vi "report page.vi"() -> (2 "This VI":refnum<vi>)   [LabVIEW 2019]
uses:
  <vilib>/addons/database/NI_Database_API.lvlib
  <vilib>/addons/database/_DB Variant To Data/Database Variant To Data.xnode
  <vilib>/addons/database/Connection.llb/DB Tools Open Connec (String).vi
  <vilib>/Utility/NIReport.llb/NI_report.lvclass
  <vilib>/Utility/NIReport.llb/Append Text Table to Report (wrap).vi
  <vilib>/Utility/miscctls.llb/LVRowAndColumnTypeDef.ctl
panel:
  out "show img error":errorcluster
  in  "show":bool
  out "Selection Start":T1
  in  "stop":bool
  out "Cancel Button 2":bool
  out "Column Header Strings[]":string[](array[string])=["pallet_num", "date_time", "Grate Bar Defect", "Curvature", "SWL_sen", "SWR_sen", "SWL_cam", "SWR_cam", "def_Type", "grtbr_situation"]
  out "error out":errorcluster
  in  "curv-sit":u16(ring) items=["normal", "critical"]
  in  "curv-sit":bool
  in  "SWR-cam":u16(ring) items=["yes", "no"]
  in  "SWR-cam":bool
  in  "SWL-cam":u16(ring) items=["yes", "no"]
  in  "SWL-cam":bool
  in  "SWR-sen":u16(ring) items=["yes", "no"]
  in  "SWR_sen":bool
  in  "SWL-sen":u16(ring) items=["yes", "no"]
  in  "SWL-sen":bool
  out "Report":string
  in  "Cancel Button":bool
  out "Time":string="2019/01/29   15:25:26"
  in  "Pallet Sit":u16(ring) items=["normal", "warning", "critical"]
  in  "Defect":u16(ring) items=["Type 1", "Type 2", "Type 3"]
  in  "Pallet Num":u16=1 min=1 max=260 step=1
  in  "Time Select":u16(ring) items=["Selected Period", "Last Day", "Last Week", "Last Month"]
  in  "From":timestamp=timestamp(3613783866.3658285 s since 1904-01-01) format="%<%X\n%d/%m/%Y>T"
  in  "Until":timestamp=timestamp(3613750200 s since 1904-01-01) format="%<%X\n%d/%m/%Y>T"
  in  "Pallet_Situation":bool
  in  "Defect Type":bool
  in  "Pallet Number 2":bool
  in  "Time 2":bool
  in  "Save Button":bool
  in  "Query":bool caption="Reset Signal"
  in  "error in":errorcluster
  out "error out 2":errorcluster
  out "Table":string[][](table)
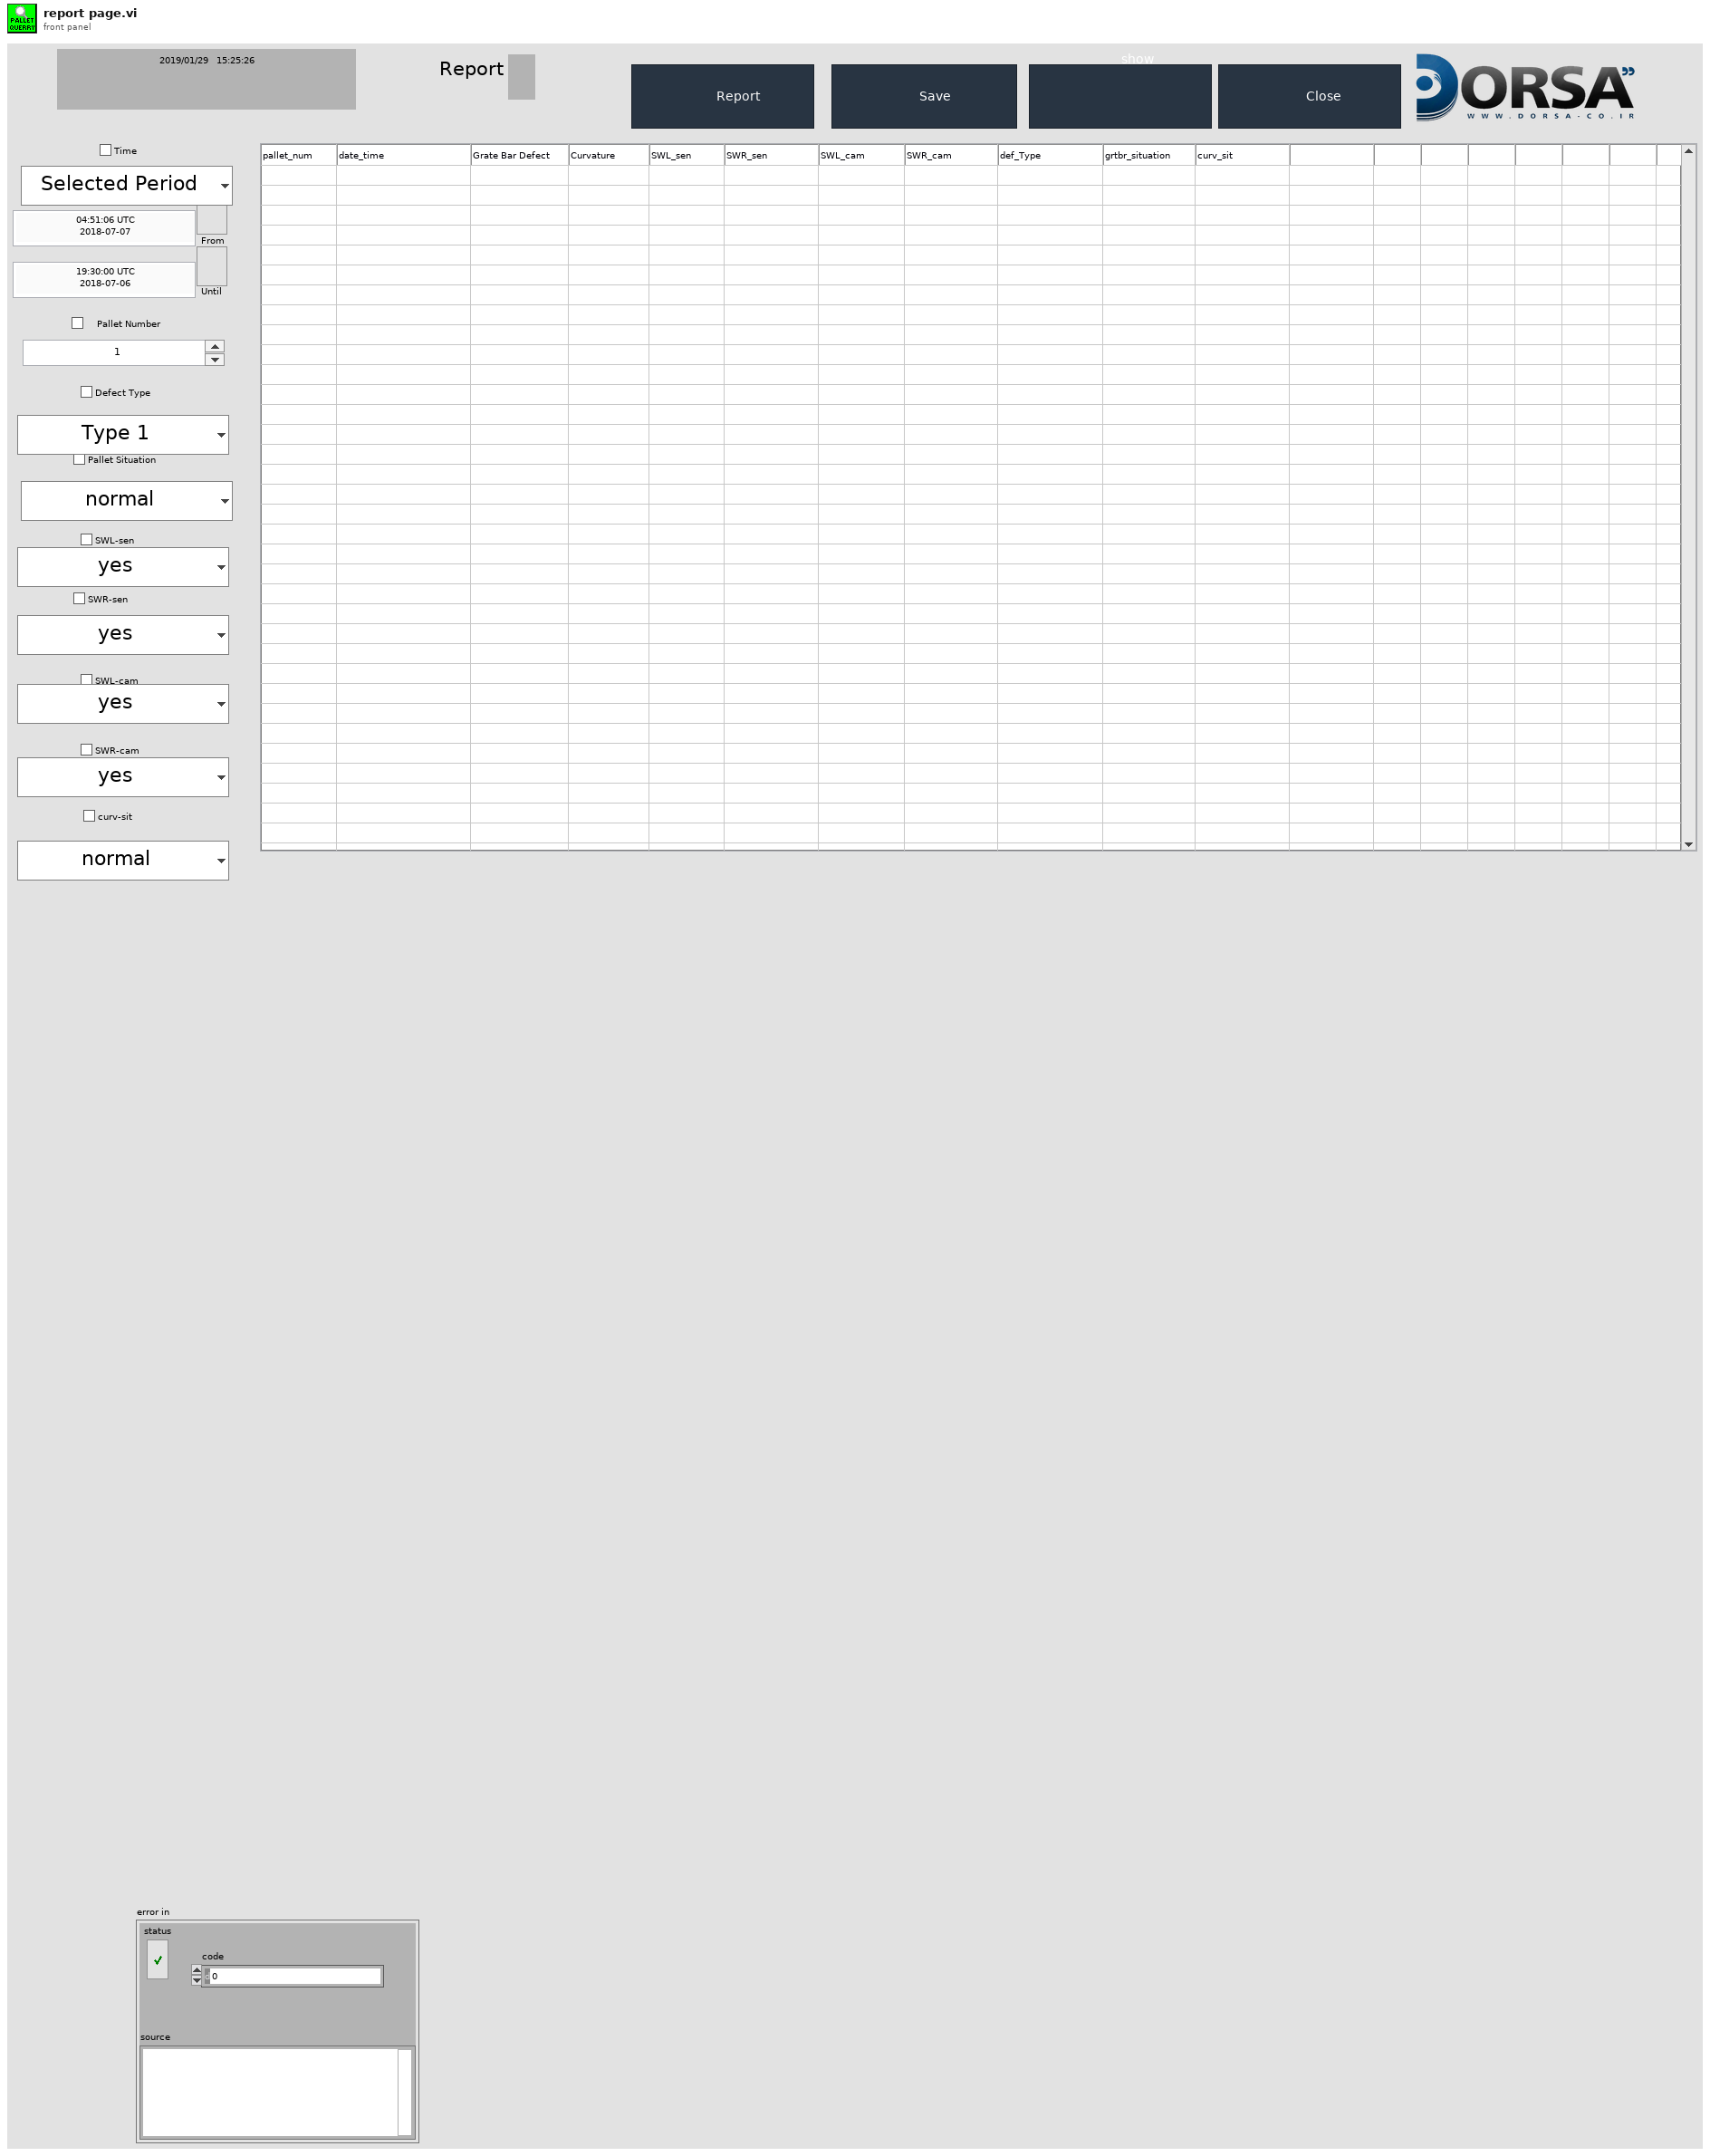
[diagram p1: front panel]
types:
  T1 = typedef "LVRowAndColumnTypeDef.ctl" = cluster{"Row":i32, "Column":i32}
  T2 = typedef "Image Type" = u32
  T3 = enum16{"Standard Report", "HTML", "Word", "Excel"}
  T4 = typedef "NI_Database_API.lvlib/Conn ObjectReference.ctl" = refnum<k1>
  T5 = typedef "IMAQ Image.ctl" = refnum<image>
  T6 = enum32{"Invalid", "Standard", "Closed", "Hidden", "Minimized", "Maximized"}
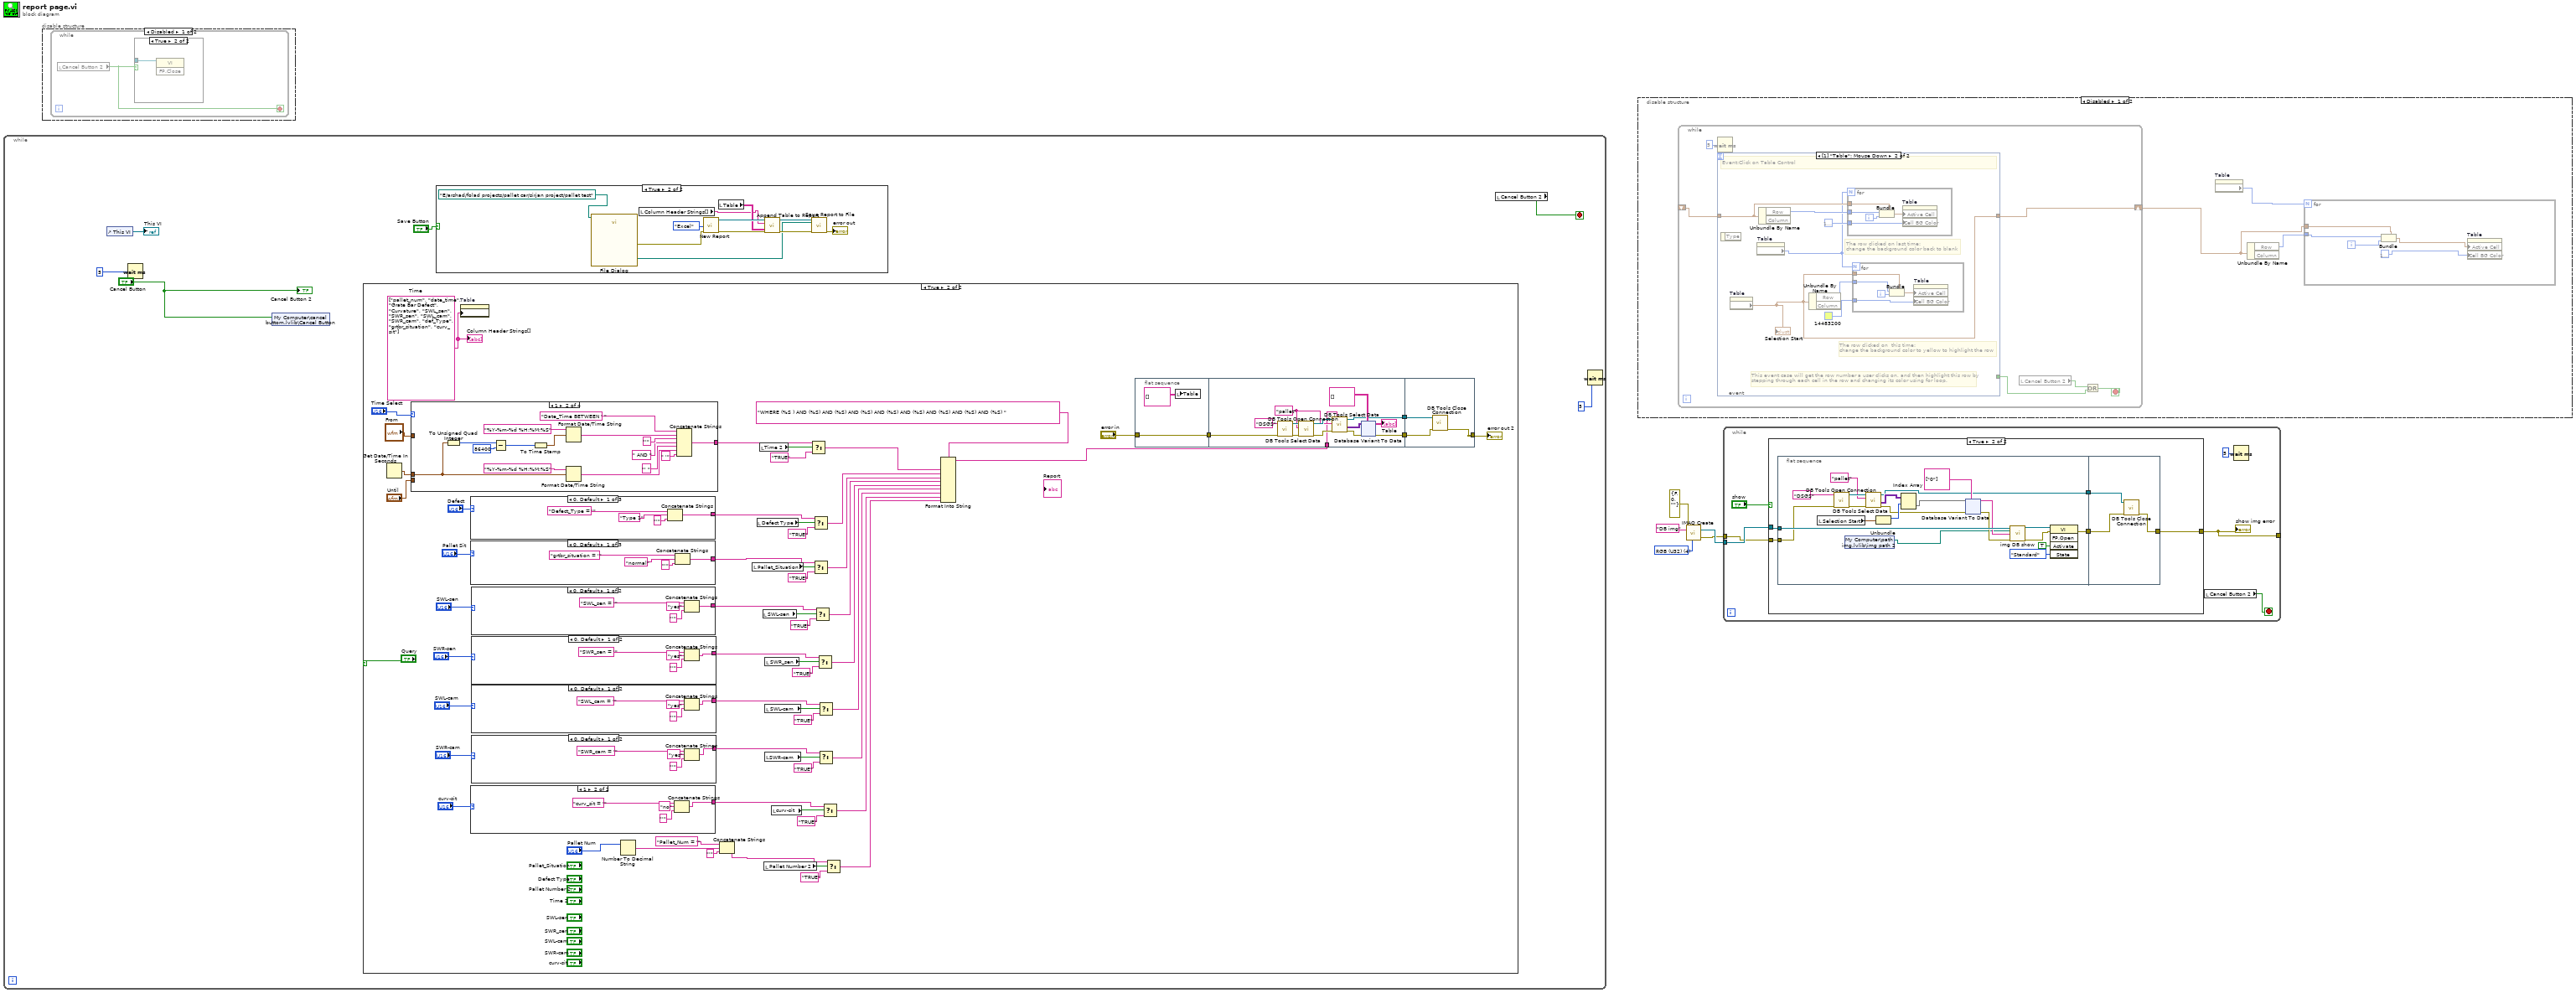
[diagram p0: block diagram]
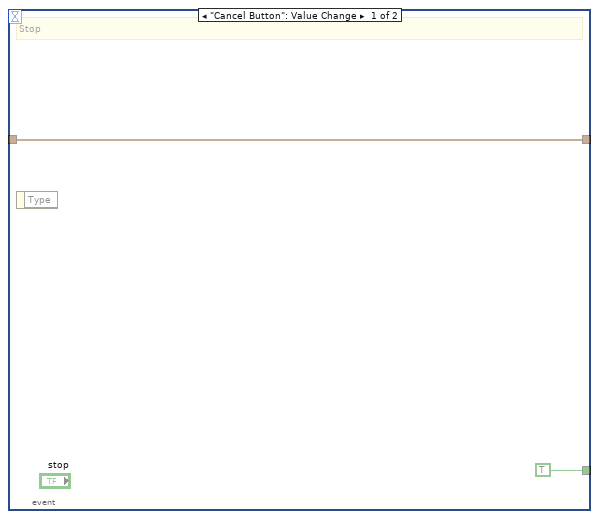
[diagram p2: hidden frame]
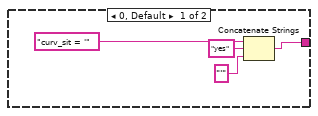
[diagram p8: hidden frame]
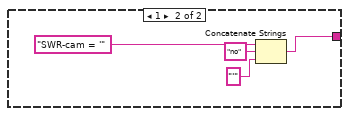
[diagram p9: hidden frame]
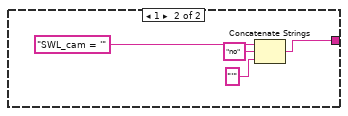
[diagram p10: hidden frame]
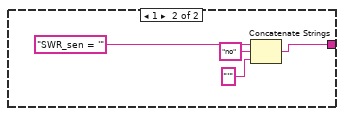
[diagram p11: hidden frame]
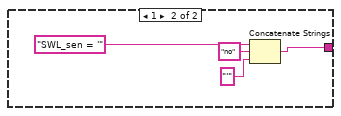
[diagram p12: hidden frame]
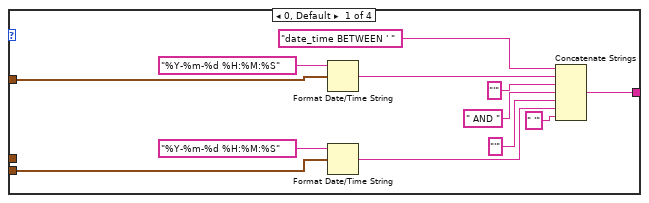
[diagram p13: hidden frame]
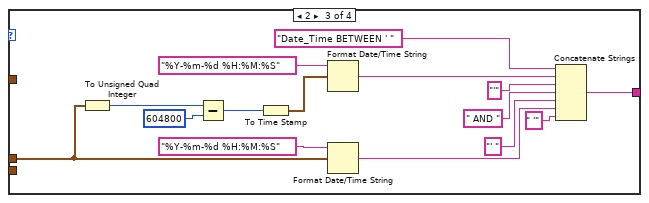
[diagram p14: hidden frame]
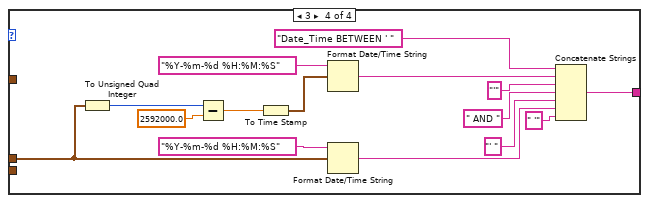
[diagram p15: hidden frame]
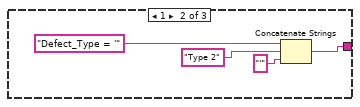
[diagram p16: hidden frame]
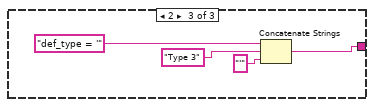
[diagram p17: hidden frame]
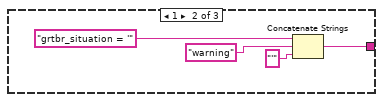
[diagram p18: hidden frame]
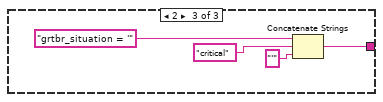
[diagram p19: hidden frame]
diagram:
  w1 = T2 4 items=["Grayscale (U8)", "Grayscale (I16)", "Grayscale (SGL)", "Complex (CSG)", "RGB (U32)", "HSL (U32)", "RGB (U64)", "Grayscale (U16)"] ("Image Type")
  n1 = while {
    stop <- w11 stop-if-true
    n2 = control-ref of="This VI"() -> (→"This VI":refnum<vi>)
    n3 = Wait (ms)(milliseconds to wait=u32 5) -> ()  [unwired: 1 out]
    n4 = shared-variable "My Computer\\cancel buttom.lvlib\\Cancel Button"("Cancel Button") -> ()  [unwired: 1 in, 1 out]
    n5 = case shown="True" "Query" {
      frame False {
      }
      frame True {
        w26 = string[] ["pallet_num", "date_time", "Grate Bar Defect", "Curvature", "SWL_sen", "SWR_sen", "SWL_cam", "SWR_cam", "def_Type", "grtbr_situation", "curv_sit"] ("Column Header Strings[]")
        n6 = Get Date/Time In Seconds() -> (seconds since 1Jan1904=w73:timestamp)
        n7 = case shown="1" "Time Select" {
          tunnel: "From" -> [w193 _ _ _]
          tunnel: "Until" -> [w191 _ _ _]
          tunnel: [w186 w200 w213 w228] -> w74
          tunnel: w73 -> [_ w198 w215 w230]
          frame 0, Default {
            n8 = Format Date/Time String(time format string (%c)="%Y-%m-%d %H:%M:%S", seconds (now)=w193) -> (date/time string=w192:string)  [unwired: 1 in]
            n9 = Format Date/Time String(time format string (%c)="%Y-%m-%d %H:%M:%S", seconds (now)=w191) -> (date/time string=w188:string)  [unwired: 1 in]
            n10 = Concatenate Strings("date_time BETWEEN ' " ("condition"), w192, "'" ("condition"), " AND " ("time format string (%c)"), "'" ("string"), w188, " '" ("string")) -> (w186:string)
          }
          frame 1 {
            n11 = To Unsigned Quad Integer(1:w198) -> (0:w210:u64)
            n12 = Subtract(x=w210, y=u64 86400) -> (x-y=w212:u64)
            n13 = To Time Stamp(1:w212) -> (0:w199:timestamp)
            n14 = Format Date/Time String(time format string (%c)="%Y-%m-%d %H:%M:%S", seconds (now)=w199) -> (date/time string=w205:string)  [unwired: 1 in]
            n15 = Format Date/Time String(time format string (%c)="%Y-%m-%d %H:%M:%S", seconds (now)=w198) -> (date/time string=w202:string)  [unwired: 1 in]
            n16 = Concatenate Strings("Date_Time BETWEEN ' " ("condition"), w205, "'" ("condition"), " AND " ("time format string (%c)"), "' " ("string"), w202, " '" ("string")) -> (w200:string)
          }
          frame 2 {
            n17 = To Unsigned Quad Integer(1:w215) -> (0:w218:u64)
            n18 = Subtract(x=w218, y=u64 604800) -> (x-y=w216:u64)
            n19 = To Time Stamp(1:w216) -> (0:w214:timestamp)
            n20 = Format Date/Time String(time format string (%c)="%Y-%m-%d %H:%M:%S", seconds (now)=w214) -> (date/time string=w223:string)  [unwired: 1 in]
            n21 = Format Date/Time String(time format string (%c)="%Y-%m-%d %H:%M:%S", seconds (now)=w215) -> (date/time string=w220:string)  [unwired: 1 in]
            n22 = Concatenate Strings("Date_Time BETWEEN ' " ("condition"), w223, "'" ("condition"), " AND " ("time format string (%c)"), "' " ("string"), w220, " '" ("string")) -> (w213:string)
          }
          frame 3 {
            n23 = To Unsigned Quad Integer(1:w230) -> (0:w232:u64)
            n24 = Subtract(x=w232, y=2592000.0) -> (x-y=w233:dbl)
            n25 = To Time Stamp(1:w233) -> (0:w229:timestamp)
            n26 = Format Date/Time String(time format string (%c)="%Y-%m-%d %H:%M:%S", seconds (now)=w229) -> (date/time string=w238:string)  [unwired: 1 in]
            n27 = Format Date/Time String(time format string (%c)="%Y-%m-%d %H:%M:%S", seconds (now)=w230) -> (date/time string=w241:string)  [unwired: 1 in]
            n28 = Concatenate Strings("Date_Time BETWEEN ' " ("condition"), w238, "'" ("condition"), " AND " ("time format string (%c)"), "' " ("string"), w241, " '" ("string")) -> (w228:string)
          }
        }
        n29 = property on="Table" class="Tbl (strict)"("Column Headers[]"=w26) -> ()  [unwired: 2 in, 2 out]
        n30 = case shown="0, Default" "Defect" {
          tunnel: [w243 w247 w251] -> w76
          frame 0, Default {
            n31 = Concatenate Strings("Defect_Type = '" ("string"), "Type 1" ("string"), "'" ("string")) -> (w243:string)
          }
          frame 1 {
            n32 = Concatenate Strings("Defect_Type = '" ("string"), "Type 2" ("string"), "'" ("string")) -> (w247:string)
          }
          frame 2 {
            n33 = Concatenate Strings("def_type = '" ("string"), "Type 3" ("string"), "'" ("string")) -> (w251:string)
          }
        }
        n34 = case shown="0, Default" "Pallet Sit" {
          tunnel: [w255 w259 w263] -> w77
          frame 0, Default {
            n35 = Concatenate Strings("grtbr_situation = '" ("string"), "normal" ("string"), "'" ("string")) -> (w255:string)
          }
          frame 1 {
            n36 = Concatenate Strings("grtbr_situation = '" ("string"), "warning" ("string"), "'" ("string")) -> (w259:string)
          }
          frame 2 {
            n37 = Concatenate Strings("grtbr_situation = '" ("string"), "critical" ("string"), "'" ("string")) -> (w263:string)
          }
        }
        n38 = case shown="1" "curv-sit" {
          tunnel: [w146 w150] -> w55
          frame 0, Default {
            n39 = Concatenate Strings("curv_sit = '" ("string"), "yes" ("string"), "'" ("string")) -> (w146:string)
          }
          frame 1 {
            n40 = Concatenate Strings("curv_sit = '" ("string"), "no" ("string"), "'" ("string")) -> (w150:string)
          }
        }
        n41 = case shown="0, Default" "SWL-sen" {
          tunnel: [w178 w182] -> w59
          frame 0, Default {
            n42 = Concatenate Strings("SWL_sen = '" ("string"), "yes" ("string"), "'" ("string")) -> (w178:string)
          }
          frame 1 {
            n43 = Concatenate Strings("SWL_sen = '" ("string"), "no" ("string"), "'" ("string")) -> (w182:string)
          }
        }
        n44 = case shown="0, Default" "SWR-sen" {
          tunnel: [w170 w174] -> w58
          frame 0, Default {
            n45 = Concatenate Strings("SWR_sen = '" ("string"), "yes" ("string"), "'" ("string")) -> (w170:string)
          }
          frame 1 {
            n46 = Concatenate Strings("SWR_sen = '" ("string"), "no" ("string"), "'" ("string")) -> (w174:string)
          }
        }
        n47 = case shown="0, Default" "SWL-cam" {
          tunnel: [w162 w166] -> w57
          frame 0, Default {
            n48 = Concatenate Strings("SWL_cam = '" ("string"), "yes" ("string"), "'" ("string")) -> (w162:string)
          }
          frame 1 {
            n49 = Concatenate Strings("SWL_cam = '" ("string"), "no" ("string"), "'" ("string")) -> (w166:string)
          }
        }
        n50 = case shown="0, Default" "SWR-cam" {
          tunnel: [w154 w158] -> w56
          frame 0, Default {
            n51 = Concatenate Strings("SWR_cam = '" ("string"), "yes" ("string"), "'" ("string")) -> (w154:string)
          }
          frame 1 {
            n52 = Concatenate Strings("SWR-cam = '" ("string"), "no" ("string"), "'" ("string")) -> (w158:string)
          }
        }
        n53 = Number To Decimal String(number="Pallet Num") -> (decimal integer string=w81:string)  [unwired: 1 in]
        n54 = Concatenate Strings("Pallet_Num = '" ("string"), w81, "'" ("string")) -> (w75:string)
        n55 = local read "Pallet_Situation"() -> (w50:bool)
        n56 = local read "Defect Type"() -> (w51:bool)
        n57 = local read "Time 2"() -> (w54:bool)
        n58 = local read "SWL-sen"() -> (w47:bool)
        n59 = local read "Pallet Number 2"() -> (w38:bool)
        n60 = local read "SWR-cam"() -> (w42:bool)
        n61 = local read "SWR_sen"() -> (w46:bool)
        n62 = local read "SWL-cam"() -> (w43:bool)
        n63 = local read "curv-sit"() -> (w39:bool)
        n64 = Select(t=w74, s=w54, f="TRUE") -> (s? t:f=w36:string)
        n65 = Select(t=w76, s=w51, f="TRUE") -> (s? t:f=w35:string)
        n66 = Select(t=w77, s=w50, f="TRUE") -> (s? t:f=w34:string)
        n67 = Select(t=w59, s=w47, f="TRUE") -> (s? t:f=w33:string)
        n68 = Select(t=w58, s=w46, f="TRUE") -> (s? t:f=w32:string)
        n69 = Select(t=w57, s=w43, f="TRUE") -> (s? t:f=w31:string)
        n70 = Select(t=w56, s=w42, f="TRUE") -> (s? t:f=w30:string)
        n71 = Select(t=w55, s=w39, f="TRUE") -> (s? t:f=w29:string)
        n72 = Select(t=w75, s=w38, f="TRUE") -> (s? t:f=w28:string)
        n73 = Format Into String(format string="WHERE (%S ) AND (%S) AND (%S) AND (%S) AND (%S) AND (%S) AND (%S) AND (%S) AND (%S) ", w36, w35, w34, w33, w32, w31, w30, w29, w28) -> (resulting string=w78:string)  [unwired: 2 in, 1 out]
        n74 = flat-sequence {
          tunnel: [w83] -> w82
          tunnel: "error in" -> [w83]
          tunnel: w82 -> [w96]
          tunnel: w78 -> [w85]
          tunnel: [w91] -> w25
          tunnel: [w86] -> w24
          tunnel: [w143] -> w71
          tunnel: w25 -> [w144]
          tunnel: w24 -> [w145]
          frame #0 {
            n75 = local write "Table"(string[][] []) -> ()
          }
          frame #1 {
            w88 = "pallet" ("table name")
            n76 = call-poly <vilib>:"DB Tools Open Connection.vi"("error in (no error)"=w96, "connection information"="DSGS" ("Database")) -> ("error out"=w95:errorcluster, "connection reference"=w94:T4)  [unwired: 6 in]
            n77 = call <vilib>:"DB Tools Select Data.vi"("error in (no error)"=w95, "table"=w88, "connection reference"=w94) -> ("error out"=w93:errorcluster, "connection reference out"=w92:T4)  [unwired: 3 in, 1 out]
            n78 = call <vilib>:"DB Tools Select Data.vi"("condition"=w85, "error in (no error)"=w93, "table"=w88, "connection reference"=w92) -> ("error out"=w98:errorcluster, "data"=w97:variant[][], "connection reference out"=w86:T4)  [unwired: 2 in]
            n79 = xnode "Database Variant To Data"("database variant"=w97, "error in (no error)"=w98, "type"=string[][] []) -> ("data"=→"Table":string[][], "error out"=w91:errorcluster)
          }
          frame #2 {
            n80 = call <vilib>:"DB Tools Close Connection.vi"("error in (no error)"=w144, "connection reference"=w145) -> ("error out"=w143:errorcluster)  [unwired: 5 in]
          }
        }
        "error out 2" <- w71
        "Column Header Strings[]" <- w26
      }
    }
    n81 = case shown="True" "Save Button" {
      frame False {
      }
      frame True {
        n82 = call "File Dialog"("start path"=path "E:/arshad/folad projects/pallet car/sirjan project/pallet test" ("report file path")) -> ("selected path"=w14:path, "error out"=w13:errorcluster)  [unwired: 11 in, 2 out]
        n83 = local read "Column Header Strings[]"() -> (w16:string[])
        n84 = call <vilib>:"New Report.vi"("report type"=T3."Excel", "error in (no error)"=w13) -> ("report out"=w22:refnum<class "NI_report.lvclass">, "error out"=w21:errorcluster)  [unwired: 12 in]
        n85 = local read "Table"() -> (w20:string[][])
        n86 = call-poly <vilib>:"Append Table to Report.vi"("report in"=w22, "column headers"=w16, "text data"=w20, "error in (no error)"=w21) -> ("report out"=w19:refnum<class "NI_report.lvclass">, "error out"=w18:errorcluster)  [unwired: 8 in, 2 out]
        n87 = call-dynamic "Save Report to File.vi"("report in"=w19, "report file path"=w14, "error in (no error)"=w18) -> ("error out"=→"error out":errorcluster)  [unwired: 11 in, 1 out]
      }
    }
    n88 = local read "Cancel Button 2"() -> (w11:bool)
    n89 = Wait (ms)(milliseconds to wait=u32 5) -> ()  [unwired: 1 out]
    "Cancel Button 2" <- "Cancel Button"
  }
  n90 = disable-structure shown="Disabled" {
    frame Disabled {
      n91 = while {
        stop <- w268 stop-if-true
        n92 = local read "Cancel Button 2"() -> (w268:bool)
        n93 = case shown="True" w268 {
          tunnel: [_ w269] -> w267
          frame False {
          }
          frame True {
            n94 = invoke class="VI" method="FP.Close"(reference=w269) -> ()  [unwired: 2 in, 3 out]
          }
        }
      }
    }
    frame Enabled {
    }
  }
  n95 = disable-structure shown="Disabled" {
    frame Disabled {
      n96 = while {
        shift-right: [w281] -> w270
        shift-left: _ -> [w282]
        stop <- w278 stop-if-true
        n97 = event shown="[1] \"Table\": Mouse Down" {
          selector: _ -> [_ _]
          dyn-events: _ -> [_ _]
          timeout: _ -> [_ _]
          tunnel: [w285 w287] -> w281
          tunnel: w282 -> [w285 w288]
          tunnel: [TRUE _] -> w279
          event "Cancel Button": Value Change {
            # "Stop"
            n98 = event-data() -> ()  [unwired: 1 in, 1 out]
          }
          event "Table": Mouse Down {
            # "This event case will get the row number a user clicks on, and then highlight this row by \nstepping through each cell in the row and changing its color using for loop."
            # "The row clicked on  this time:\nchange the background color to yellow to highlight the row"
            # "The row clicked on last time:\nchange the background color back to blank"
            # "Event:Click on Table Control"
            n99 = event-data() -> ()  [unwired: 1 in, 1 out]
            n100 = property on="Table" class="Tbl (strict)"() -> ("Selection Start"=w287:T1)  [unwired: 2 in, 2 out]
            "Selection Start" <- w287
            n101 = property on="Table" class="Tbl (strict)"() -> ("Number of Columns"=w286:u32)  [unwired: 2 in, 2 out]
            n102 = Unbundle By Name(w288) -> ("Row"=w290:i32)  [unwired: 1 out]
            n103 = Unbundle By Name(w287) -> ("Row"=w291:i32)  [unwired: 1 out]
            n104 = for {
              N: w286 -> [_]
              tunnel: u32 16777226 -> [w293]
              tunnel: w288 -> [w297]
              tunnel: w290 -> [w296]
              i -> [w295]
              n105 = Bundle(cluster=w297, "Row"=w296, "Column"=w295) -> (w294:T1)
              n106 = property on="Table" class="Tbl (strict)"("Active Cell"=w294, "Cell BG Color"=w293) -> ()  [unwired: 2 in, 2 out]
            }
            n107 = for {
              N: w286 -> [_]
              tunnel: u32 14483200 -> [w298]
              tunnel: w287 -> [w302]
              tunnel: w291 -> [w301]
              i -> [w300]
              n108 = Bundle(cluster=w302, "Row"=w301, "Column"=w300) -> (w299:T1)
              n109 = property on="Table" class="Tbl (strict)"("Active Cell"=w299, "Cell BG Color"=w298) -> ()  [unwired: 2 in, 2 out]
            }
          }
        }
        n110 = Wait (ms)(milliseconds to wait=u32 5) -> ()  [unwired: 1 out]
        n111 = local read "Cancel Button 2"() -> (w280:bool)
        n112 = Or(x=w280, y=w279) -> (x .or. y?=w278:bool)
      }
      n113 = property on="Table" class="Tbl (strict)"() -> ("Number of Columns"=w271:u32)  [unwired: 2 in, 2 out]
      n114 = Unbundle By Name(w270) -> ("Row"=w272:i32)  [unwired: 1 out]
      n115 = for {
        N: w271 -> [_]
        tunnel: w272 -> [w276]
        tunnel: w270 -> [w277]
        i -> [w275]
        n116 = Bundle(cluster=w277, "Row"=w276, "Column"=w275) -> (w273:T1)
        n117 = property on="Table" class="Tbl (strict)"("Active Cell"=w273, "Cell BG Color"=u32 16777226) -> ()  [unwired: 2 in, 2 out]
      }
    }
    frame Enabled {
    }
  }
  n118 = call "IMAQ Create"("Image Name"="DB img", "Image Type"=w1, "error in (no error)"=errorcluster {"status"=FALSE, "code"=0, "source"=""}) -> ("New Image"=w5:T5, "error out"=w4:errorcluster)  [unwired: 2 in]
  n119 = while {
    tunnel: w5 -> [w308]
    tunnel: w4 -> [w307]
    tunnel: [w303] -> _
    stop <- w305 stop-if-true
    n120 = case shown="True" "show" {
      tunnel: w308 -> [_ w314]
      tunnel: w307 -> [w309 w313]
      tunnel: [w309 w312] -> w303
      frame False {
      }
      frame True {
        n121 = flat-sequence {
          tunnel: w314 -> [w327]
          tunnel: w313 -> [w325]
          tunnel: [w317] -> w311
          tunnel: [w315] -> w310
          tunnel: [w374] -> w312
          tunnel: w311 -> [w375]
          tunnel: w310 -> [w376]
          frame #0 {
            n122 = local read "Selection Start"() -> (w329:T1)
            n123 = call-poly <vilib>:"DB Tools Open Connection.vi"("error in (no error)"=w325, "connection information"="DSGS" ("Database")) -> ("error out"=w324:errorcluster, "connection reference"=w334:T4)  [unwired: 6 in]
            n124 = shared-variable "My Computer\\path img.lvlib\\img path 2"() -> (w316:path)  [unwired: 1 in, 1 out]
            n125 = call <vilib>:"DB Tools Select Data.vi"("error in (no error)"=w324, "table"="pallet" ("table name"), "connection reference"=w334) -> ("error out"=w323:errorcluster, "data"=w332:variant[][], "connection reference out"=w315:T4)  [unwired: 3 in]
            n126 = Unbundle(w329) -> ("Row"=w328:i32)  [unwired: 1 out]
            n127 = Index Array(array=w332, index (row)=w328) -> (element=w331:variant[])  [unwired: 1 in]
            n128 = xnode "Database Variant To Data"("database variant"=w331, "error in (no error)"=w323, "type"=string[] ["0"] ("columns")) -> ("data"=w326:string[], "error out"=w322:errorcluster)
            n129 = call "img DB show.vi"("Image 2"=w327, "File Path"=w316, "data"=w326, "error in (no error)"=w322) -> ("This VI"=w321:refnum<vi>, "error out"=w318:errorcluster)  [unwired: 10 in]
            n130 = invoke class="VI" method="FP.Open"(reference=w321, error in=w318, "Activate"=TRUE ("Activate?"), "State"=T6."Standard") -> (error out=w317:errorcluster)  [unwired: 1 in, 4 out]
          }
          frame #1 {
            n131 = call <vilib>:"DB Tools Close Connection.vi"("error in (no error)"=w375, "connection reference"=w376) -> ("error out"=w374:errorcluster)  [unwired: 5 in]
          }
        }
      }
    }
    "show img error" <- w303
    n132 = local read "Cancel Button 2"() -> (w305:bool)
    n133 = Wait (ms)(milliseconds to wait=u32 5) -> ()  [unwired: 1 out]
  }
